vi "CustomPID_v4.1_Testing.vi"(0 "PID Tuning Parameters":T1={"Kp"=0.1, "Ki"=0.1, "Kd"=0.1, "N-Diff"=10, "N-Int"=20, "Int Error Window"=0.5, "Max Ouput"=1.0, "Min Output"=-1.0, "Square Derivative"=FALSE, "N-Prop"=1} {"N-Prop" min=1; "Int Error Window" min=0.0; "N-Int" min=2; "N-Diff" min=2; "Kd" min=0.0; "Ki" min=0.0; "Kp" min=0.0}, 1 "Goal":dbl(slide) scale=-1.0..1.0, 2 "Process Variable":dbl(slide) scale=-1.0..1.0, 3 "Custom Error Calculation":dbl(slide) scale=-1.0..1.0, 7 "Reset on Goal Change ?":bool, 9 "Use Custom Error Calculation ?":bool, 12 "Reinit":bool) -> (4 "Command":dbl format="%_4g", 6 "Is Reset":bool, 8 "Current Error":dbl format="%_4g", 15 "Controller Summary":T2(graph))   [LabVIEW 2019]
doc: "Brief PID Description:\n\nA good mechanical analogy for a PID algorithm is a spring-mass system with a viscous damper \n(https://ccrma.stanford.edu/CCRMA/Courses/150/img35.gif). The proportional term is the \"spring,\" it has the strongest influence when the robot system is furthest from its goal. The derivative term is the damping coefficient, it's what allows the system to stop oscillating and reach it's goal. The integral term mostly comes into play if the robot has been been trying to move for a lengthy amount of time but still isn't able to reach it's goal (this is referred to as steady-state error).\n\nRecommended Tuning Procedure:\n\n1) You may want to restrict the Max and Min Output parameters more than [-1, 1] during initial tuning to avoid damaging the system.\n2) Carefully increase the Kp term from 0.0001 until the system starts moving.\n3) If the system is going the wrong direction, you may need to negate the Command.\n4) Continue inceasing Kp until the system oscillates about the Goal.\n5) Carefully increase Kd from 0.0001 until the system's response is sufficiently damped (i.e. until the oscillation is mitigated).\n6) Carefully increase Ki from 0.0001 to reduce the steady-state error (SSE) (if any).\n7) Adjust N-Diff if necessary (minimum of 2). Increasing N-Diff will reduce the effects of sensor (Process Variable) noise on the \nderivative term but will increase the lag on that component. You may also want to add a filter to Process Variable data.\n8) Adjust N-Int if necessary (minimum of 2). Increasing N-Int may help the system overcome SSE but may also increase integrator wind-up. It will also increase the lag for that component.\n9) Another way to reduce integrator wind-up is to set the Integral Error Window. The Intergral term will only be used if the magnitude of the error is less than the specified window.\n10) You may need to adjust Kp, Ki, and Kd after adjusting N-Diff and N-Int. \n\nAdditional Notes:\n\n1) Make sure that execution type for all instances of this VI are set to \"preallocated clone reentrant execution.\"\n2) Several parts of this VI were inspired by a PID algorithm written by Dr. Ira Hill at the University of Florida.\n3) If you have any questions, feel free to contact me at lrscime.alpha@gmail.coms"
uses:
  <vilib>/Analysis/6fits.llb/Curve Fitting Criteria.ctl
  <vilib>/Analysis/4window.llb/Exponential Window (DBL).vi
  <vilib>/Analysis/NI_AALPro.lvlib
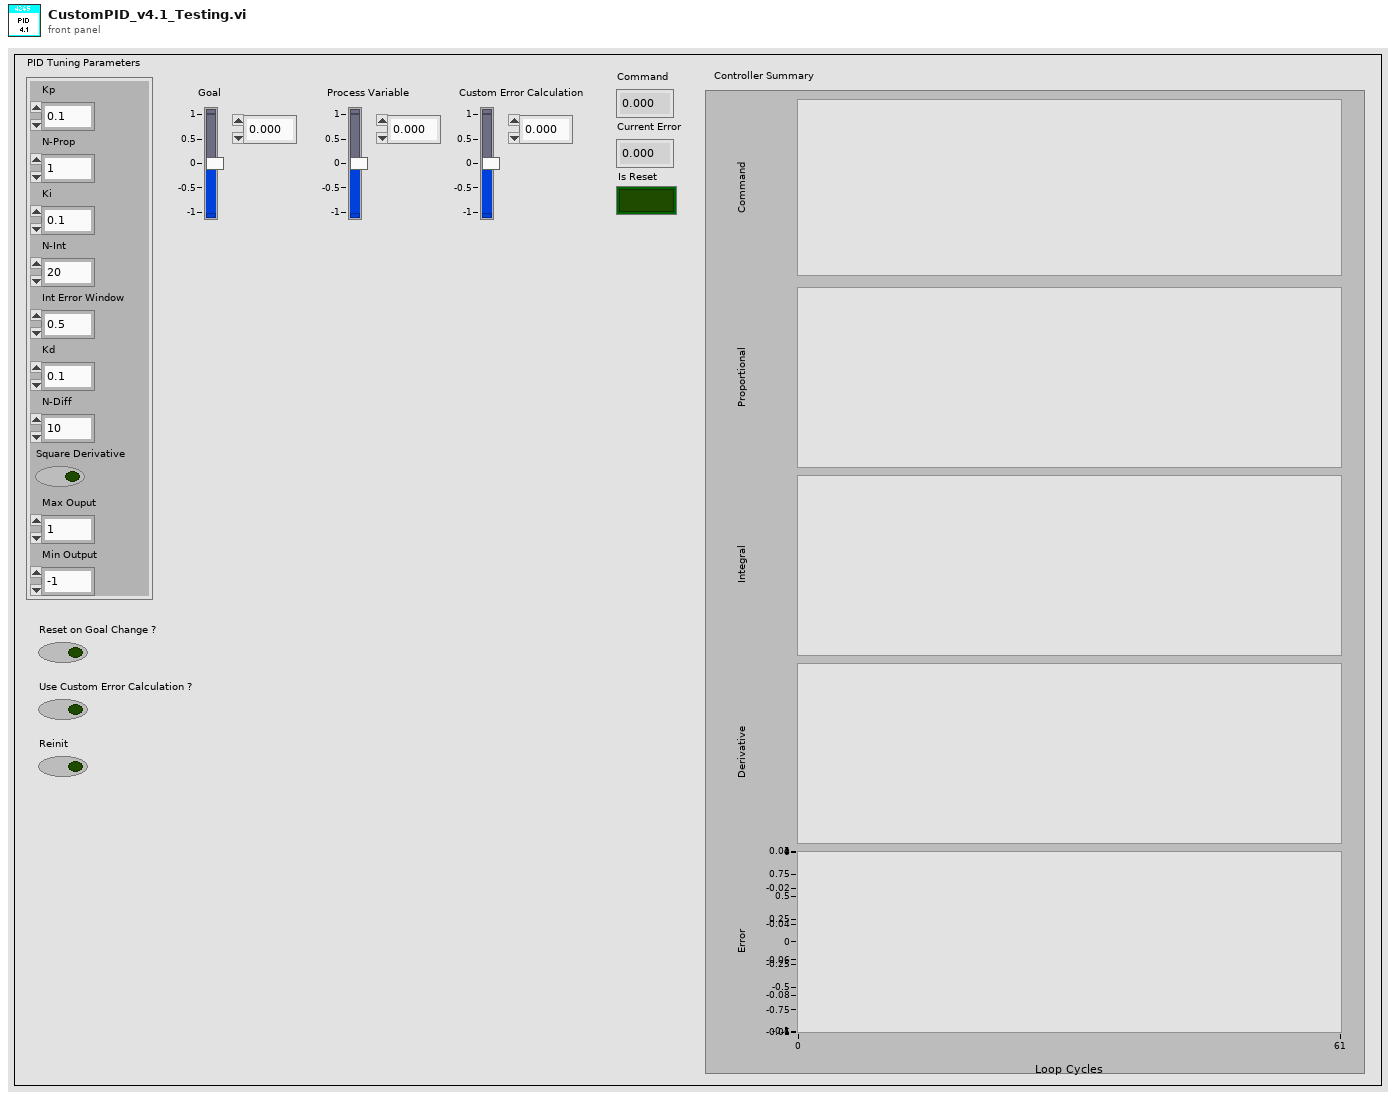
[diagram p1: front panel]
types:
  T1 = cluster{"Kp":dbl, "Ki":dbl, "Kd":dbl, "N-Diff":i32, "N-Int":i32, "Int Error Window":dbl, "Max Ouput":dbl, "Min Output":dbl, "Square Derivative":bool, "N-Prop":i32}
  T2 = cluster{"Command":dbl, "Proportional":dbl, "Integral":dbl, "Derivative":dbl, "Goal":dbl}
  T3 = cluster{"Command":dbl, "Proportional":dbl, "Integral":dbl, "Derivative":dbl, "Error":dbl}
  T4 = typedef "NI_AALPro.lvlib/Curve Fitting Criteria.ctl" = u16
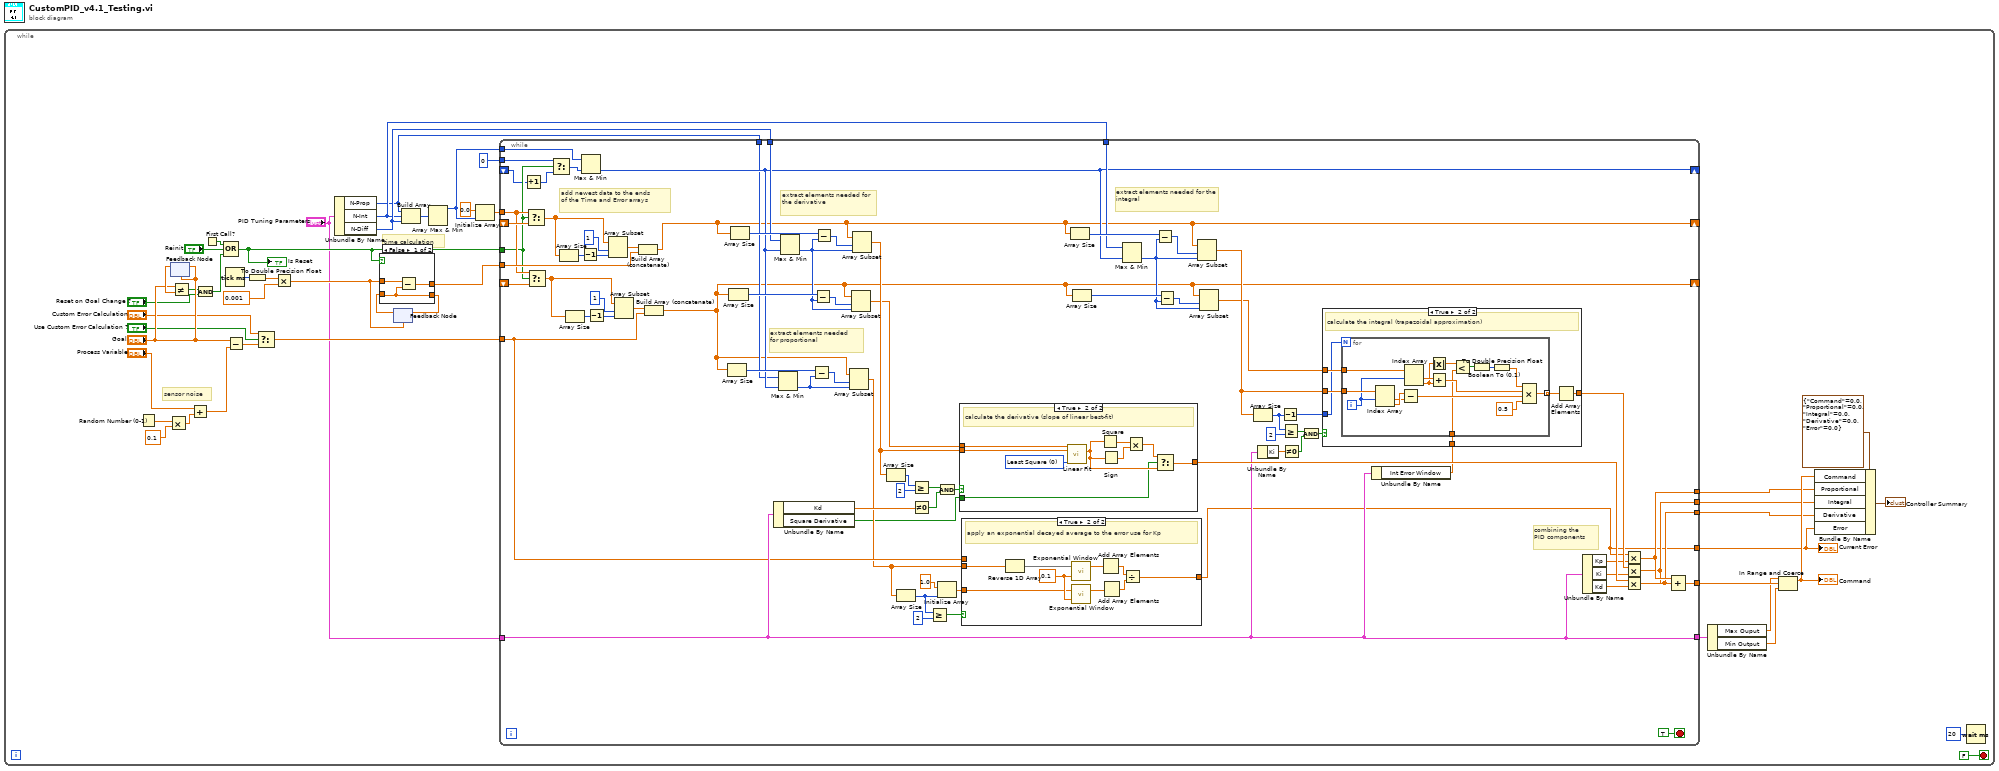
[diagram p0: block diagram]
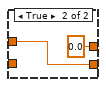
[diagram p2: hidden frame]
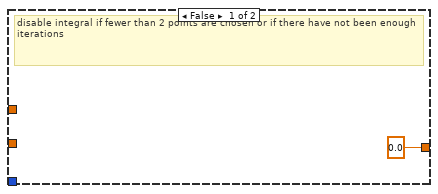
[diagram p4: hidden frame]
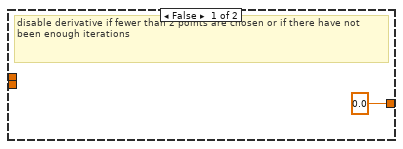
[diagram p5: hidden frame]
diagram:
  n1 = while {
    stop <- FALSE stop-if-true
    # "sensor noise"
    # "time calculation"
    n2 = Random Number (0-1)() -> (number: 0 to 1=w10:dbl)
    n3 = Multiply(x=w10, y=0.1) -> (x*y=w8:dbl)
    n4 = feedback #1("Goal") -> (w41:dbl)
    n5 = feedback-in #1("Goal") -> ()
    n6 = Not Equal?(x="Goal", y=w41) -> (x != y?=w24:bool)
    n7 = Add(x="Process Variable", y=w8) -> (x+y=w6:dbl)
    n8 = And(x=w24, y="Reset on Goal Change ?") -> (x .and. y?=w34:bool)
    n9 = First Call?() -> (First Call?: T/F=w45:bool)
    n10 = Compound Arithmetic op=OR(w45, "Reinit", w34) -> (w35:bool)
    "Is Reset" <- w35
    n11 = Tick Count (ms)() -> (millisecond timer value=w40:u32)
    n12 = Subtract(x="Goal", y=w6) -> (x-y=w22:dbl)
    n13 = To Double Precision Float(number=w40) -> (double precision float=w39:dbl)
    n14 = Select(t="Custom Error Calculation", s="Use Custom Error Calculation ?", f=w22) -> (s? t:f=w21:dbl)
    n15 = Multiply(x=w39, y=0.001) -> (x*y=w33:dbl)
    n16 = Unbundle By Name("PID Tuning Parameters") -> ("N-Prop"=w1:i32, "N-Int"=w4:i32, "N-Diff"=w5:i32)
    n17 = feedback #2(w33) -> (w36:dbl)
    n18 = case shown="False" w35 {
      tunnel: w33 -> [w49 w51]
      tunnel: [w47 w51] -> w37
      tunnel: [w48 0.0] -> w27
      tunnel: w36 -> [w47 _]
      frame False {
        n19 = Subtract(x=w49, y=w47) -> (x-y=w48:dbl)
      }
      frame True {
      }
    }
    n20 = feedback-in #2(w37) -> ()
    n21 = Build Array(w1, w4, w5) -> (w3:i32[])
    n22 = Array Max & Min(array=w3) -> (max value=w2:i32)  [unwired: 3 out]
    n23 = Initialize Array(0.0 ("element"), w2) -> (w43:dbl[])
    n24 = while {
      tunnel: [w127] -> w46
      tunnel: w21 -> [w65]
      shift-right: [w55] -> _
      shift-left: _ -> [w104]
      tunnel: w27 -> [w122]
      shift-right: [w54] -> _
      shift-left: _ -> [w101]
      tunnel: w35 -> [w93]
      tunnel: w43 -> [w102]
      tunnel: [w64] -> w18
      tunnel: [w97] -> w31
      tunnel: [w96] -> w30
      tunnel: [w95] -> w29
      tunnel: 0 -> [w94]
      shift-right: [w57] -> _
      shift-left: _ -> [w91]
      tunnel: w2 -> [w88]
      tunnel: w4 -> [w78]
      tunnel: w5 -> [w77]
      tunnel: "PID Tuning Parameters" -> [w70]
      tunnel: [w70] -> w15
      tunnel: w1 -> [w56]
      stop <- TRUE stop-if-true
      # "extract elements needed\nfor proportional"
      # "combining the\nPID components"
      # "add newest data to the ends\nof the Time and Error arrays"
      # "extract elements needed for the integral"
      # "extract elements needed for the derivative"
      n25 = Increment(x=w91) -> (x+1=w92:i32)
      n26 = Select(t=w102, s=w93, f=w104) -> (s? t:f=w103:dbl[])
      n27 = Select(t=w102, s=w93, f=w101) -> (s? t:f=w100:dbl[])
      n28 = Select(t=w94, s=w93, f=w92) -> (s? t:f=w89:i32)
      n29 = Array Size(array=w103) -> (size(s)=w125:i32)
      n30 = Array Size(array=w100) -> (size(s)=w120:i32)
      n31 = Decrement(x=w125) -> (x-1=w124:i32)
      n32 = Max & Min(x=w88, y=w89) -> (min(x,y)=w57:i32)  [unwired: 1 out]
      n33 = Decrement(x=w120) -> (x-1=w119:i32)
      n34 = Array Subset(array=w103, index=1, length=w124) -> (w123:dbl[])
      n35 = Array Subset(array=w100, index=1, length=w119) -> (w118:dbl[])
      n36 = Build Array (concatenate)(w123, w122) -> (w55:dbl[])
      n37 = Build Array (concatenate)(w118, w65) -> (w54:dbl[])
      n38 = Array Size(array=w54) -> (size(s)=w60:i32)
      n39 = Array Size(array=w54) -> (size(s)=w114:i32)
      n40 = Array Size(array=w55) -> (size(s)=w117:i32)
      n41 = Unbundle By Name(w70) -> ("Kd"=w76:dbl, "Square Derivative"=w52:bool)
      n42 = Max & Min(x=w56, y=w57) -> (min(x,y)=w58:i32)  [unwired: 1 out]
      n43 = Max & Min(x=w77, y=w57) -> (min(x,y)=w90:i32)  [unwired: 1 out]
      n44 = Subtract(x=w60, y=w58) -> (x-y=w59:i32)
      n45 = Subtract(x=w114, y=w90) -> (x-y=w115:i32)
      n46 = Subtract(x=w117, y=w90) -> (x-y=w116:i32)
      n47 = Array Subset(array=w54, index=w59, length=w58) -> (w53:dbl[])
      n48 = Array Subset(array=w54, index=w115, length=w90) -> (w67:dbl[])
      n49 = Array Subset(array=w55, index=w116, length=w90) -> (w113:dbl[])
      n50 = Array Size(array=w113) -> (size(s)=w68:i32)
      n51 = Array Size(array=w53) -> (size(s)=w62:i32)
      n52 = Greater Or Equal?(x=w68, y=2) -> (x >= y?=w87:bool)
      n53 = Not Equal To 0?(x=w76) -> (x != 0?=w85:bool)
      n54 = Greater Or Equal?(x=w62, y=2) -> (x >= y?=w61:bool)
      n55 = Initialize Array(1.0 ("element"), w62) -> (w66:dbl[])
      n56 = Compound Arithmetic op=AND(w87, w85) -> (w86:bool)
      n57 = case shown="True" w86 {
        tunnel: w67 -> [_ w169]
        tunnel: w113 -> [_ w170]
        tunnel: [0.0 w165] -> w98
        tunnel: w52 -> [_ w163]
        frame False {
          # "disable derivative if fewer than 2 points are chosen or if there have not been enough iterations"
        }
        frame True {
          w171 = T4 0 items=["Least Square", "Least Absolute Residual", "Bisquare"] ("method")
          # "calculate the derivative (slope of linear best-fit)"
          n58 = call <vilib>:"Linear Fit.vi"("Y"=w169, "X"=w170, "method"=w171) -> ("slope"=w164:dbl)  [unwired: 8 in, 4 out]
          n59 = Square(x=w164) -> (x^2=w167:dbl)
          n60 = Sign(1:w164) -> (0:w168:dbl)
          n61 = Multiply(x=w167, y=w168) -> (x*y=w166:dbl)
          n62 = Select(t=w166, s=w163, f=w164) -> (s? t:f=w165:dbl)
        }
      }
      n63 = case shown="True" w61 {
        tunnel: w53 -> [_ w132]
        tunnel: w66 -> [_ w131]
        tunnel: w65 -> [w129 _]
        tunnel: [w129 w130] -> w64
        frame False {
          # "disable error averaging if fewer than 2 points are chosen or if there have not been enough iterations"
        }
        frame True {
          w137 = 0.1 ("final value")
          # "apply an exponential decayed average to the error use for Kp"
          n64 = Reverse 1D Array(array=w132) -> (reversed array=w133:dbl[])
          n65 = call-poly <vilib>:"Exponential Window.vi"("final value"=w137, "X"=w133) -> ("Windowed X"=w138:dbl[])  [unwired: 1 out]
          n66 = call-poly <vilib>:"Exponential Window.vi"("final value"=w137, "X"=w131) -> ("Windowed X"=w136:dbl[])  [unwired: 1 out]
          n67 = Add Array Elements(numeric array=w138) -> (sum=w135:dbl)
          n68 = Add Array Elements(numeric array=w136) -> (sum=w134:dbl)
          n69 = Divide(x=w135, y=w134) -> (x/y=w130:dbl)
        }
      }
      n70 = Array Size(array=w55) -> (size(s)=w111:i32)
      n71 = Array Size(array=w54) -> (size(s)=w109:i32)
      n72 = Max & Min(x=w78, y=w57) -> (min(x,y)=w84:i32)  [unwired: 1 out]
      n73 = Subtract(x=w111, y=w84) -> (x-y=w110:i32)
      n74 = Subtract(x=w109, y=w84) -> (x-y=w108:i32)
      n75 = Array Subset(array=w55, index=w110, length=w84) -> (w105:dbl[])
      n76 = Array Subset(array=w54, index=w108, length=w84) -> (w99:dbl[])
      n77 = Array Size(array=w105) -> (size(s)=w83:i32)
      n78 = Unbundle By Name(w70) -> ("Ki"=w75:dbl)
      n79 = Decrement(x=w83) -> (x-1=w82:i32)
      n80 = Greater Or Equal?(x=w83, y=2) -> (x >= y?=w81:bool)
      n81 = Not Equal To 0?(x=w75) -> (x != 0?=w79:bool)
      n82 = Compound Arithmetic op=AND(w81, w79) -> (w80:bool)
      n83 = Unbundle By Name(w70) -> ("Int Error Window"=w74:dbl)
      n84 = case shown="True" w80 {
        tunnel: [0.0 w140] -> w106
        tunnel: w105 -> [_ w145]
        tunnel: w99 -> [_ w144]
        tunnel: w74 -> [_ w143]
        tunnel: w82 -> [_ w142]
        frame False {
          # "disable integral if fewer than 2 points are chosen or if there have not been enough iterations"
        }
        frame True {
          # "calculate the integral (trapezoidal approximation)"
          n85 = for {
            N: w142 -> [_]
            tunnel: w145 -> [w161]
            tunnel: w144 -> [w155]
            tunnel: w143 -> [w148]
            tunnel: [w147] -> w141 mode=indexing
            i -> [w156]
            n86 = Index Array(array=w161, index #1=w156) -> (element #1=w159:dbl, element #2=w160:dbl)  [unwired: 1 in]
            n87 = Subtract(x=w160, y=w159) -> (x-y=w158:dbl)
            n88 = Index Array(array=w155, index #1=w156) -> (element #1=w153:dbl, element #2=w146:dbl)  [unwired: 1 in]
            n89 = Absolute Value(x=w146) -> (abs(x)=w152:dbl)
            n90 = Add(x=w153, y=w146) -> (x+y=w154:dbl)
            n91 = Less?(x=w152, y=w148) -> (x < y?=w151:bool)
            n92 = Boolean To (0,1)(Boolean=w151) -> (0, 1=w150:i16)
            n93 = To Double Precision Float(number=w150) -> (double precision float=w149:dbl)
            n94 = Compound Arithmetic op=MULTIPLY(w149, w154, w158, 0.5 ("value")) -> (w147:dbl)
          }
          n95 = Add Array Elements(numeric array=w141) -> (sum=w140:dbl)
        }
      }
      n96 = Unbundle By Name(w70) -> ("Kp"=w73:dbl, "Ki"=w72:dbl, "Kd"=w71:dbl)
      n97 = Multiply(x=w64, y=w73) -> (x*y=w97:dbl)
      n98 = Multiply(x=w106, y=w72) -> (x*y=w96:dbl)
      n99 = Multiply(x=w98, y=w71) -> (x*y=w95:dbl)
      n100 = Compound Arithmetic op=ADD(w97, w96, w95) -> (w127:dbl)
    }
    "Current Error" <- w18
    n101 = Unbundle By Name(w15) -> ("Max Ouput"=w14:dbl, "Min Output"=w13:dbl)
    n102 = In Range and Coerce(upper limit=w14, x=w46, lower limit=w13) -> (coerced(x)=w32:dbl)  [unwired: 1 out]
    "Command" <- w32
    n103 = Bundle By Name(cluster=T3 {"Command"=0.0, "Proportional"=0.0, "Integral"=0.0, "Derivative"=0.0, "Error"=0.0} ("input cluster"), "Command"=w32, "Proportional"=w31, "Integral"=w30, "Derivative"=w29, "Error"=w18) -> (→"Controller Summary":T3)
    n104 = Wait (ms)(milliseconds to wait=u32 20) -> ()  [unwired: 1 out]
  }
